vi "Unflatten.vi"(8 "error in":errorcluster, 10 "Buffer":u8[](array[numeric]) format="%.0x") -> (0 "error out":errorcluster, 2 "Data":T1)   [LabVIEW 2020, in "BoolData.lvlib"]
uses:
  BoolData.lvlib
  Data.ctl
  lv-protoc/LV-Proto/Wire Decode Varint I32.vi
  lv-protoc/LV-Proto/Extract Varint Bytes.vi
  lv-protoc/LV-Proto/LV-Proto.lvlib
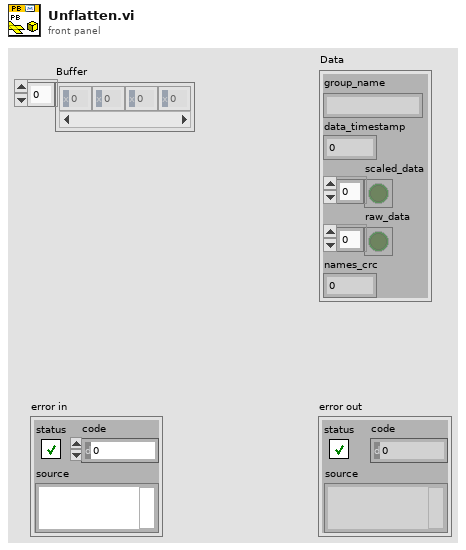
[diagram p1: front panel]
types:
  T1 = typedef "BoolData.lvlib/Data.ctl" = cluster{"group_name":string, "data_timestamp":i64, "scaled_data":bool[], "raw_data":bool[], "names_crc":u32}
  T2 = typedef "LV-Proto.lvlib/Wire Type.ctl" = enum8{"VARINT", "I64", "LEN", "SGROUP (Deprecated)", "EGROUP (Deprecated)", "I32"}
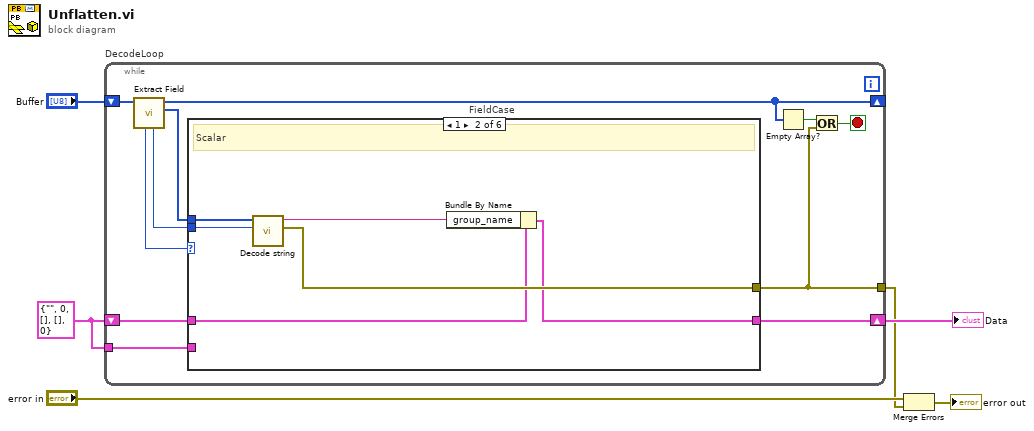
[diagram p0: block diagram]
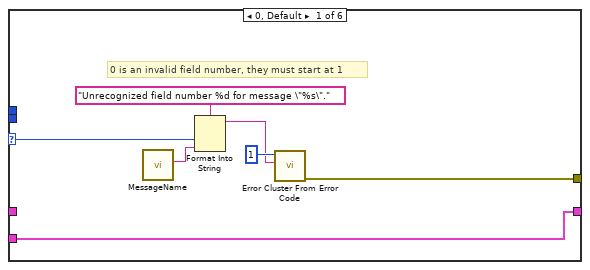
[diagram p2: hidden frame]
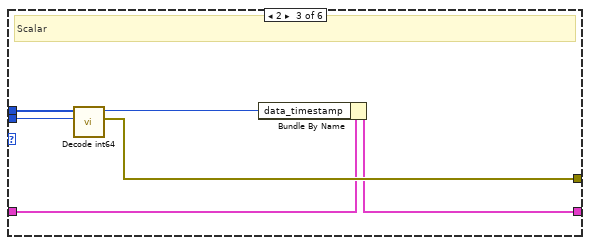
[diagram p3: hidden frame]
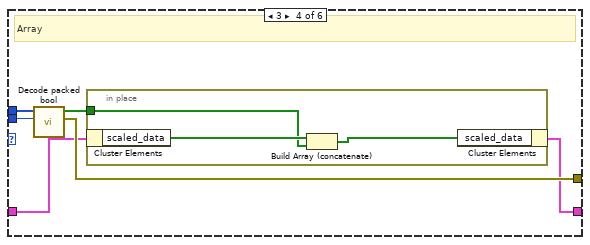
[diagram p4: hidden frame]
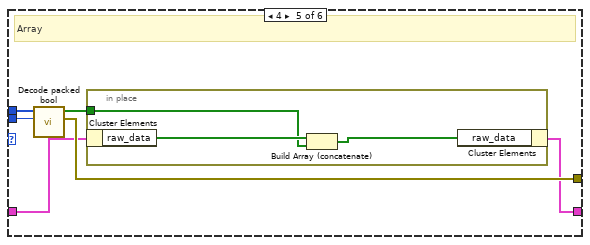
[diagram p5: hidden frame]
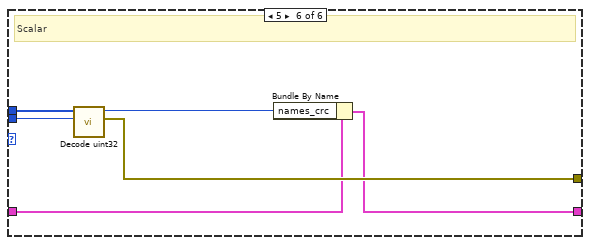
[diagram p6: hidden frame]
diagram:
  w4 = T1 {"group_name"="", "data_timestamp"=0, "scaled_data"=[], "raw_data"=[], "names_crc"=0} ("Data")
  n1 = while "DecodeLoop" {
    shift-right: [w16] -> _
    shift-left: "Buffer" -> [w17]
    shift-right: [w9] -> w5
    shift-left: w4 -> [w15]
    tunnel: [w8] -> w2
    tunnel: w4 -> [w7]
    stop <- w11 stop-if-true
    n2 = call "Extract Field.vi"("Buffer in"=w17) -> ("Field Data"=w10:u8[], "Buffer"=w16:u8[], "Wire Type"=w13:T2, "Field Number"=w14:i32)  [unwired: 7 in]
    n3 = case "FieldCase" shown="1" w14 {
      selector: w14 -> [w23 _ _ _ _ _]
      tunnel: w15 -> [_ w26 w32 w39 w48 w56]
      tunnel: w13 -> [_ w28 w34 w40 w49 w58]
      tunnel: w10 -> [_ w29 w35 w41 w50 w59]
      tunnel: [w19 w25 w31 w38 w47 w55] -> w9
      tunnel: [w20 w30 w36 w42 w51 w60] -> w8
      tunnel: w7 -> [w19 _ _ _ _ _]
      frame 0, Default {
        # "0 is an invalid field number, they must start at 1"
        n4 = call "MessageName.vi"() -> ("MessageName"=w18:string)  [unwired: 11 in]
        n5 = Format Into String(format string="Unrecognized field number %d for message \"%s\".", w23, w18) -> (resulting string=w21:string)  [unwired: 2 in, 1 out]
        n6 = call <vilib>:"Error Cluster From Error Code.vi"("error message (\"\")"=w21, "error code (0)"=1) -> ("error out"=w20:errorcluster)  [unwired: 7 in]
      }
      frame 1 {
        # "Scalar"
        n7 = call "Decode string.vi"("Wire Type"=w28, "Data"=w29) -> ("error out"=w30:errorcluster, "string"=w27:string)  [unwired: 8 in]
        n8 = Bundle By Name(cluster=w26, "group_name"=w27) -> (w25:T1)
      }
      frame 2 {
        # "Scalar"
        n9 = call "Decode int64.vi"("Wire Type"=w34, "Data"=w35) -> ("error out"=w36:errorcluster, "int64"=w33:i64)  [unwired: 8 in]
        n10 = Bundle By Name(cluster=w32, "data_timestamp"=w33) -> (w31:T1)
      }
      frame 3 {
        # "Array"
        n11 = call "Decode packed bool.vi"("Wire Type"=w40, "Data"=w41) -> ("error out"=w42:errorcluster, "bool"=w37:bool[])  [unwired: 8 in]
        n12 = in-place {
          in-place-border: w37 -> [w43]
          n13 = in-place-cluster #1(w39) -> ("scaled_data"=w45:bool[])
          n14 = Build Array (concatenate)(w45, w43) -> (w44:bool[])
          n15 = in-place-cluster #1("scaled_data"=w44) -> (w38:T1)
        }
      }
      frame 4 {
        # "Array"
        n16 = call "Decode packed bool.vi"("Wire Type"=w49, "Data"=w50) -> ("error out"=w51:errorcluster, "bool"=w46:bool[])  [unwired: 8 in]
        n17 = in-place {
          in-place-border: w46 -> [w52]
          n18 = in-place-cluster #2(w48) -> ("raw_data"=w54:bool[])
          n19 = Build Array (concatenate)(w54, w52) -> (w53:bool[])
          n20 = in-place-cluster #2("raw_data"=w53) -> (w47:T1)
        }
      }
      frame 5 {
        # "Scalar"
        n21 = call "Decode uint32.vi"("Wire Type"=w58, "Data"=w59) -> ("error out"=w60:errorcluster, "uint32"=w57:u32)  [unwired: 8 in]
        n22 = Bundle By Name(cluster=w56, "names_crc"=w57) -> (w55:T1)
      }
    }
    n23 = Empty Array?(array=w16) -> (empty?=w12:bool)
    n24 = Or(x=w12, y=w8) -> (x .or. y?=w11:bool)
  }
  "Data" <- w5
  n25 = Merge Errors("error in", w2) -> (→"error out":errorcluster)
